vi "compare_vi_to_disk.vi"   [LabVIEW 2009]
uses:
  <userlib>/_OpenG.lib/file/file.llb/Valid Path - Traditional__ogtk.vi
  <userlib>/_OpenG.lib/file/file.llb/Convert File Extension (Path)__ogtk.vi
types:
  T1 = typedef "VIMemory VI info.ctl" = cluster{"Project":string, "ComputingNode":string, "VI Name":string, "App Refnum":refnum<vi>}
  T2 = cluster{"VI Attributes":bool, "Front Panel":bool, "FP pos/size":bool, "Block Diagram":bool, "BD cosmetic":bool, "BD pos/size":bool}
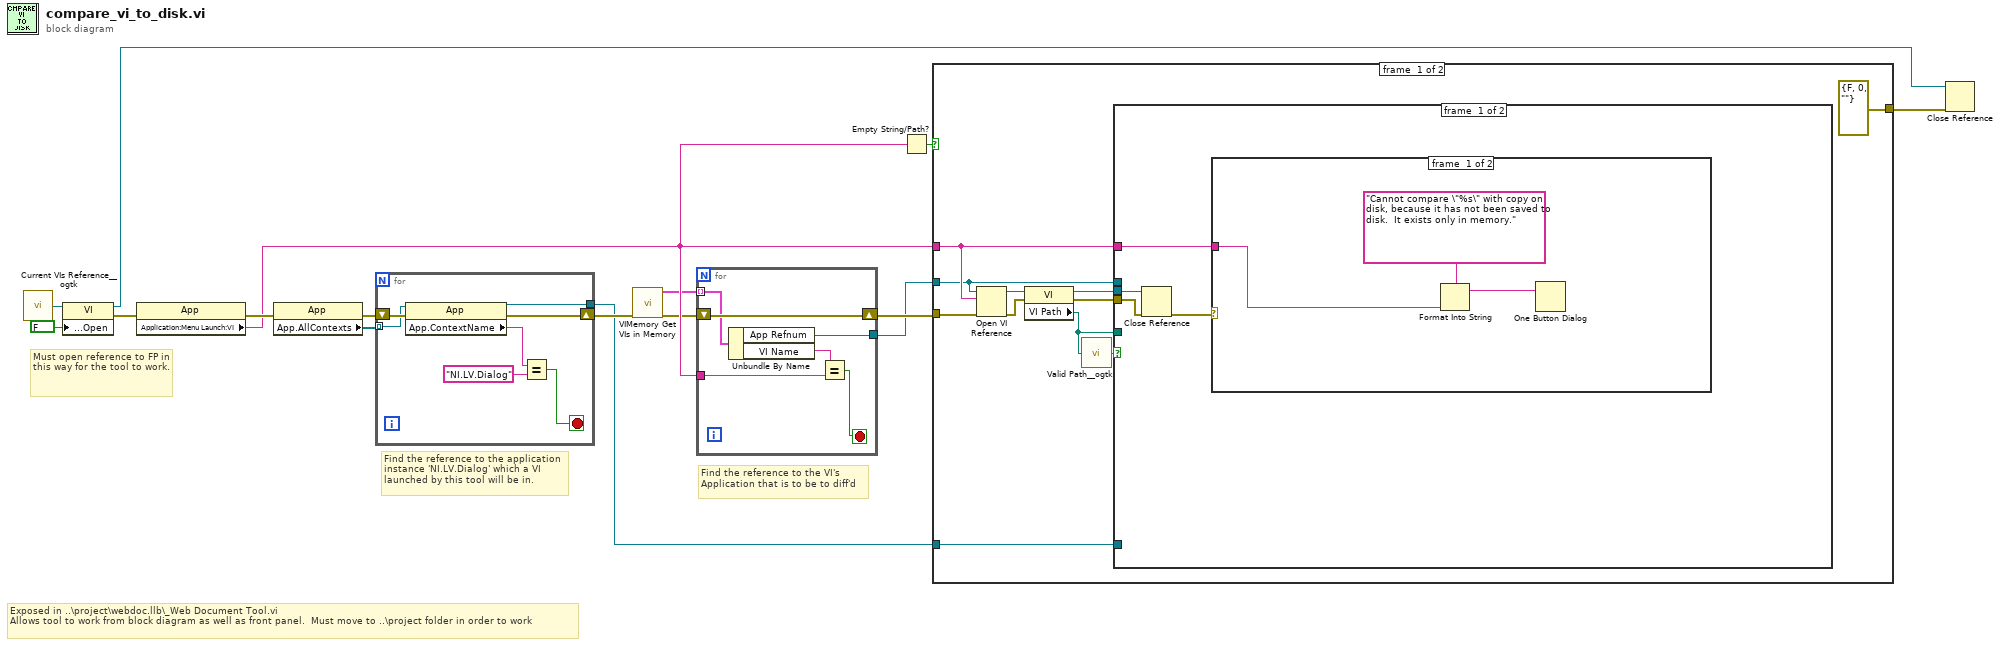
[diagram p0: block diagram]
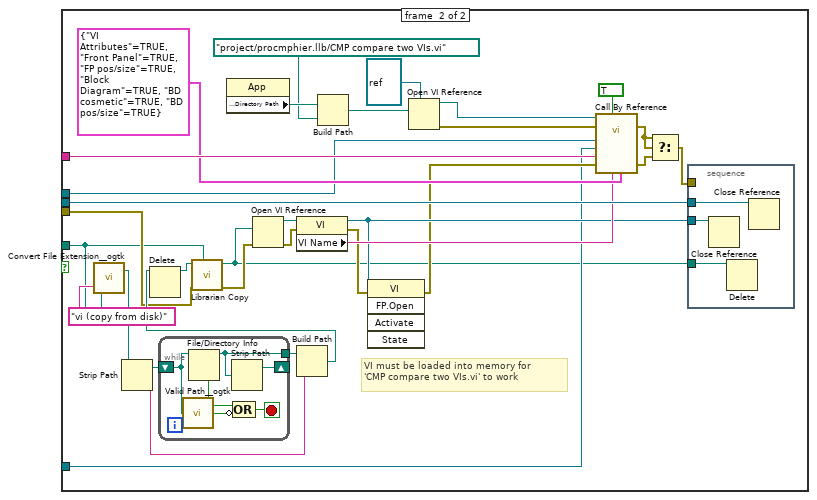
[diagram p3: hidden frame]
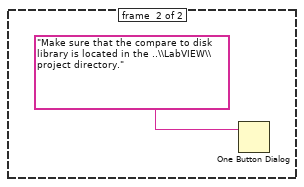
[diagram p4: hidden frame]
diagram:
  # "Must open reference to FP in this way for the tool to work."
  # "Find the reference to the VI's Application that is to be to diff'd"
  # "Find the reference to the application instance 'NI.LV.Dialog' which a VI launched by this tool will be in."
  # "Exposed in ..\\project\\webdoc.llb\\_Web Document Tool.vi\nAllows tool to work from block diagram as well as front panel.  Must move to ..\\project folder in order to work"
  n1 = call <userlib>:"Current VIs Reference__ogtk.vi"() -> ("Current VI's reference"=w1:refnum<vi>)  [unwired: 5 in]
  n2 = property class="VI"(reference=w1, "Front Panel Window:Open"=FALSE) -> (reference out=w3:refnum<vi>, error out=w4:errorcluster)  [unwired: 1 in]
  n3 = property class="App"(error in=w4) -> (error out=w12:errorcluster, "Application:Menu Launch:VI"=w10:string)  [unwired: 1 in, 1 out]
  n4 = property class="App"(error in=w12) -> (error out=w14:errorcluster, "App.AllContexts"=w13:refnum<vi>[])  [unwired: 1 in, 1 out]
  n5 = for {
    shift-right: [w22] -> w11
    shift-left: w14 -> [w23]
    tunnel: w13 -> [w19] mode=indexing
    tunnel: [w20] -> w7
    stop <- w17 stop-if-true
    n6 = property class="App"(reference=w19, error in=w23) -> (reference out=w20:refnum<vi>, error out=w22:errorcluster, "App.ContextName"=w21:string)
    n7 = Equal?(x=w21, y="NI.LV.Dialog") -> (x = y?=w17:bool)
  }
  n8 = call <vilib>:"VIMemory Get VIs in Memory.vi"("error in (no error)"=w11) -> ("error out"=w9:errorcluster, "VIs in memory"=w8:T1[])  [unwired: 9 in]
  n9 = for {
    shift-right: [w29] -> w15
    shift-left: w9 -> [w29]
    tunnel: w10 -> [w28]
    tunnel: w8 -> [w26] mode=indexing
    tunnel: [w25] -> w6
    stop <- w24 stop-if-true
    n10 = Unbundle By Name(w26) -> ("App Refnum"=w25:refnum<vi>, "VI Name"=w27:string)
    n11 = Equal?(x=w27, y=w28) -> (x = y?=w24:bool)
  }
  n12 = Empty String/Path?(string/path=w10) -> (empty?=w16:bool)
  n13 = case shown="False" w16 {
    tunnel: w10 -> [w38 _]
    tunnel: w15 -> [w35 _]
    tunnel: w7 -> [w34 _]
    tunnel: w6 -> [w33 _]
    tunnel: [errorcluster {"status"=FALSE, "code"=0, "source"=""} ("s? t:f") _] -> w2
    frame #0 {
      n14 = Open VI Reference(application reference (local)=w33, vi path=w38, error in (no error)=w35) -> (vi reference=w40:refnum<vi>, error out=w39:errorcluster)  [unwired: 3 in]
      n15 = property class="VI"(reference=w40, error in=w39) -> (reference out=w37:refnum<vi>, error out=w36:errorcluster, "VI Path"=w32:path)
      n16 = call-poly <userlib>:"Valid Path__ogtk.vi"("path"=w32) -> ("valid"=w31:bool)
      n17 = case shown="True" w31 {
        tunnel: w38 -> [w41 w68]
        tunnel: w32 -> [_ w49]
        tunnel: w37 -> [w44 w73]
        tunnel: w36 -> [w43 w52]
        tunnel: w33 -> [_ w55]
        tunnel: w34 -> [_ w56]
        frame #0 {
          n18 = Close Reference(reference=w44, error in (no error)=w43) -> (error out=w42:errorcluster)
          n19 = case shown="No Error" w42 {
            tunnel: w41 -> [w45 _]
            frame #0 {
              n20 = Format Into String(format string="Cannot compare \"%s\" with copy on disk, because it has not been saved to disk.  It exists only in memory." ("message"), w45) -> (resulting string=w46:string)  [unwired: 2 in, 1 out]
              n21 = One Button Dialog(message=w46) -> ()  [unwired: 1 in, 1 out]
            }
            frame #1 {
            }
          }
        }
        frame #1 {
          # "VI must be loaded into memory for\n'CMP compare two VIs.vi' to work"
          n22 = call-poly <userlib>:"Convert File Extension__ogtk.vi"("new ending (none)"="vi (copy from disk)", "file name"=w49) -> ("new filename"=w53:path)  [unwired: 1 out]
          n23 = Strip Path(path=w53) -> (stripped path=w72:path, name=w70:string)
          n24 = while "Strip Path to Directory\n(enables EXE install)" {
            shift-left: w72 -> [w80]
            shift-right: [w84] -> _
            tunnel: [w85] -> w71
            stop <- w82 stop-if-true
            n25 = call-poly <userlib>:"Valid Path__ogtk.vi"("path"=w80) -> ("valid"=w81:bool)
            n26 = File/Directory Info(path=w80) -> (path out=w85:path, directory=w83:bool)  [unwired: 1 in, 5 out]
            n27 = Strip Path(path=w85) -> (stripped path=w84:path)  [unwired: 1 out]
            n28 = Compound Arithmetic op=OR(w83, invert w81) -> (w82:bool)
          }
          n29 = property class="App"() -> ("Application:Directory Path"=w79:path)  [unwired: 2 in, 2 out]
          n30 = Build Path(base path=w71, name or relative path=w70) -> (appended path=w69:path)
          n31 = Delete(path (use dialog)=w69) -> (deleted path=w48:path)  [unwired: 4 in, 2 out]
          n32 = call <vilib>:"Librarian Copy.vi"("source"=w49, "error in (no error)"=w52, "destination"=w48) -> ("error out"=w51:errorcluster, "dup destination"=w50:path)  [unwired: 7 in]
          n33 = Open VI Reference(vi path=w50, error in (no error)=w51) -> (vi reference=w75:refnum<vi>, error out=w74:errorcluster)  [unwired: 4 in]
          n34 = property class="VI"(reference=w75, error in=w74) -> (reference out=w59:refnum<vi>, error out=w58:errorcluster, "VI Name"=w60:string)
          n35 = Build Path(base path=w79, name or relative path=path "project/procmphier.llb/CMP compare two VIs.vi") -> (appended path=w77:path)
          n36 = invoke class="VI" method="FP.Open"(reference=w59, error in=w58) -> (error out=w57:errorcluster)  [unwired: 3 in, 4 out]
          n37 = Open VI Reference(type specifier VI Refnum (for type only)=refnum<vi> refnum ("VI Refnum"), vi path=w77) -> (vi reference=w62:refnum<vi>, error out=w65:errorcluster)  [unwired: 4 in]
          n38 = call-by-ref "?"(reference=w62, error in=w65, "CompareOptions"=T2 {"VI Attributes"=TRUE, "Front Panel"=TRUE, "FP pos/size"=TRUE, "Block Diagram"=TRUE, "BD cosmetic"=TRUE, "BD pos/size"=TRUE} ("Compare Options"), "VIName 2"=w60, "Interactive?"=TRUE ("Interactive (F)"), 8:"error in (no error)"=w57, "VIName 1"=w68, "AppRef 2"=w56, "AppRef 1"=w55) -> (error out=w66:errorcluster, 0:"error out"=w67:errorcluster)  [unwired: 2 in, 3 out]
          n39 = Select(t=w66, s=w66, f=w67) -> (s? t:f=w76:errorcluster)
          n40 = stacked-sequence {
            tunnel: w76 -> [_]
            tunnel: w50 -> [w88]
            tunnel: w73 -> [w87]
            tunnel: w59 -> [w86]
            frame #0 {
              n41 = Close Reference(reference=w86) -> ()  [unwired: 1 in, 1 out]
              n42 = Delete(path (use dialog)=w88) -> ()  [unwired: 4 in, 3 out]
              n43 = Close Reference(reference=w87) -> ()  [unwired: 1 in, 1 out]
            }
          }
        }
      }
    }
    frame #1 {
      n44 = One Button Dialog(message="Make sure that the compare to disk library is located in the ..\\LabVIEW\\project directory.") -> ()  [unwired: 1 in, 1 out]
    }
  }
  n45 = Close Reference(reference=w3, error in (no error)=w2) -> ()  [unwired: 1 out]
